vi "Test Array to Set.vi"() -> ()   [LabVIEW 2020]
uses:
  944aec28-58bb-4328-96b7-70fcfdaad198.vi
  944aec28-58bb-4328-96b7-70fcfdaad198.vi/7c7783df-fd5a-49d9-9b7a-63cc9fb0e4e5.vi
  <vilib>/addons/_JKI Toolkits/Caraya/classes/Assert/Assert.lvclass
panel:
  out "error out":errorcluster
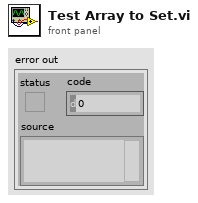
[diagram p1: front panel]
types:
  T1 = set{cluster{"Name":i32, "bool":bool, "string":string}}
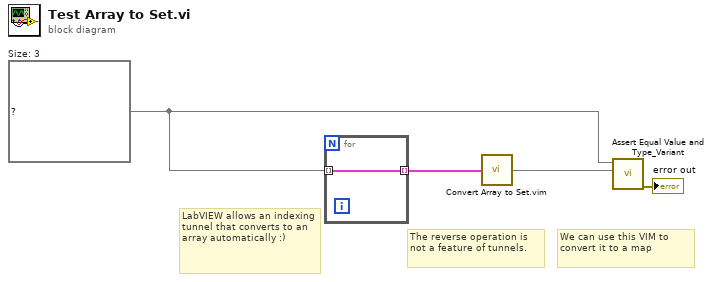
[diagram p0: block diagram]
diagram:
  w1 = T1 {{"Name"=0, "bool"=FALSE, "string"="zero"}, {"Name"=1, "bool"=TRUE, "string"="one"}, {"Name"=2, "bool"=FALSE, "string"="two"}}  # Size: 3
  # "We can use this VIM to convert it to a map"
  # "The reverse operation is not a feature of tunnels."
  # "LabVIEW allows an indexing tunnel that converts to an array automatically :)"
  n1 = for {
    tunnel: [w5] -> w4 mode=indexing
    tunnel: w1 -> [w5] mode=indexing
  }
  n2 = call "Convert Array to Set.vim"("elements"=w4) -> ("set"=w3:T1)  [unwired: 6 in]
  n3 = call <vilib>:"Assert Equal Value and Type_Variant.vi"("Y"=w3, "X"=w1) -> ("error out"=→"error out":errorcluster)  [unwired: 9 in]
